vi "resetConsoleUi.vi"(8 "error in (no error)":errorcluster, 10 "reference":refnum<vi>, 11 "Handler.UserEvent.Console in":refnum<class "Handler.UserEvent.Console.lvclass">) -> (0 "error out":errorcluster, 3 "Handler.UserEvent.Console out":refnum<class "Handler.UserEvent.Console.lvclass">)   [LabVIEW 2017, in "Error Log.lvlib" / "Handler.UserEvent.Console.lvclass"]
uses:
  Handler.UserEvent.Console.lvclass
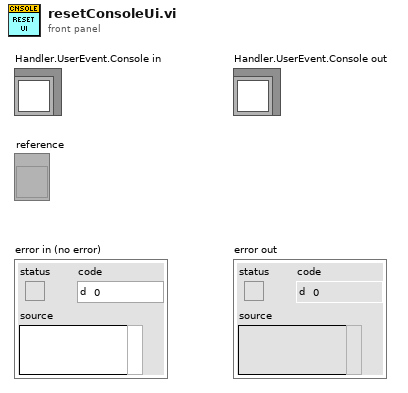
[diagram p1: front panel]
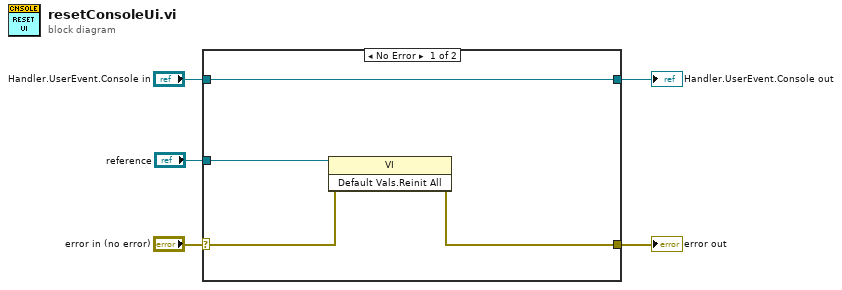
[diagram p0: block diagram]
diagram:
  n1 = case shown="No Error" "error in (no error)" {
    selector: "error in (no error)" -> [w9 w11]
    tunnel: [w8 w11] -> w4
    tunnel: [w7 w10] -> w2
    tunnel: "Handler.UserEvent.Console in" -> [w7 w10]
    tunnel: "reference" -> [w6 _]
    frame No Error {
      n2 = invoke class="VI" method="Default Vals.Reinit All"(reference=w6, error in=w9) -> (error out=w8:errorcluster)  [unwired: 1 in, 2 out]
    }
    frame Error {
    }
  }
  "error out" <- w4
  "Handler.UserEvent.Console out" <- w2
